vi "CS SQL Server.sql read.vi"(3 "error in (no error)":errorcluster, 4 "object":string, 5 "Data Source":string) -> (0 "error out":errorcluster, 1 "Class":string, 2 "query results":string[][](table))   [LabVIEW 2014, in "CS SQL Server.lvlib"]
doc: "This VI retrieves data associated with the BaseProcess attribute data from a DataBase via SQL (tested with MS Access).\n\nLicense Agreement:\n\nCopyright (C)\nGesellschaft für Schwerionenforschung, GSI\nPlanckstr. 1\n64291 Darmstadt\nGermany\n\nContact: D.Beck@gsi.de \n\nThis program is free software; you can redistribute it and/or modify it under the terms of the \nGNU General Public License as published by the Free Software Foundation; either version 2 of the license, or (at your option) any later version.\n\nThis program is distributed in the hope that it will be useful, but WITHOUT ANY WARRANTY; without even the implied warranty of MERCHANTABILITY or FITNESS FOR A PARTICULAR PURPOSE. See the GNU General License for more details (http://www.gnu.org).\n\nGesellschaft für Schwerionenforschung, GSI\nPlanckstr. 1, 64291 Darmstadt, Germany\nFor all questions and ideas contact: M.Richter@gsi.de, K.Poppensieker, H.Brand@gsi.de or D.Beck@gsi.de.\nLast update: 20-JUN-2002"
uses:
  CS SQL Server.lvlib
  <vilib>/addons/database/Recordset.llb/Rec Destroy - Connection.vi
  <vilib>/addons/database/Recordset.llb/Rec Fetch Recordset Data (R).vi
  <vilib>/addons/database/Connection.llb/Conn Execute.vi
  <vilib>/addons/database/Connection.llb/DB Tools Open Connec (String).vi
  <vilib>/addons/database/_DB Variant To Data/Database Variant To Data.xnode
  <vilib>/addons/database/NI_Database_API.lvlib
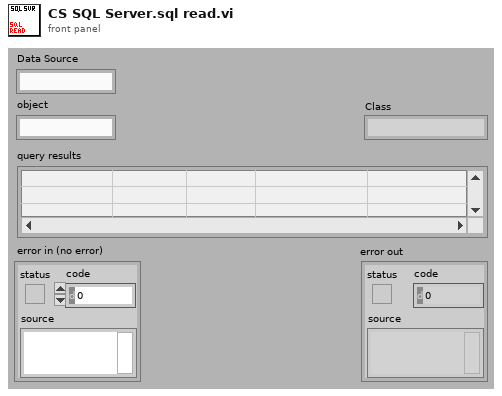
[diagram p1: front panel]
types:
  T1 = typedef "NI_Database_API.lvlib/Conn ObjectReference.ctl" = refnum<k1>
  T2 = typedef "NI_Database_API.lvlib/Rec ObjectReference.ctl" = refnum<k1>
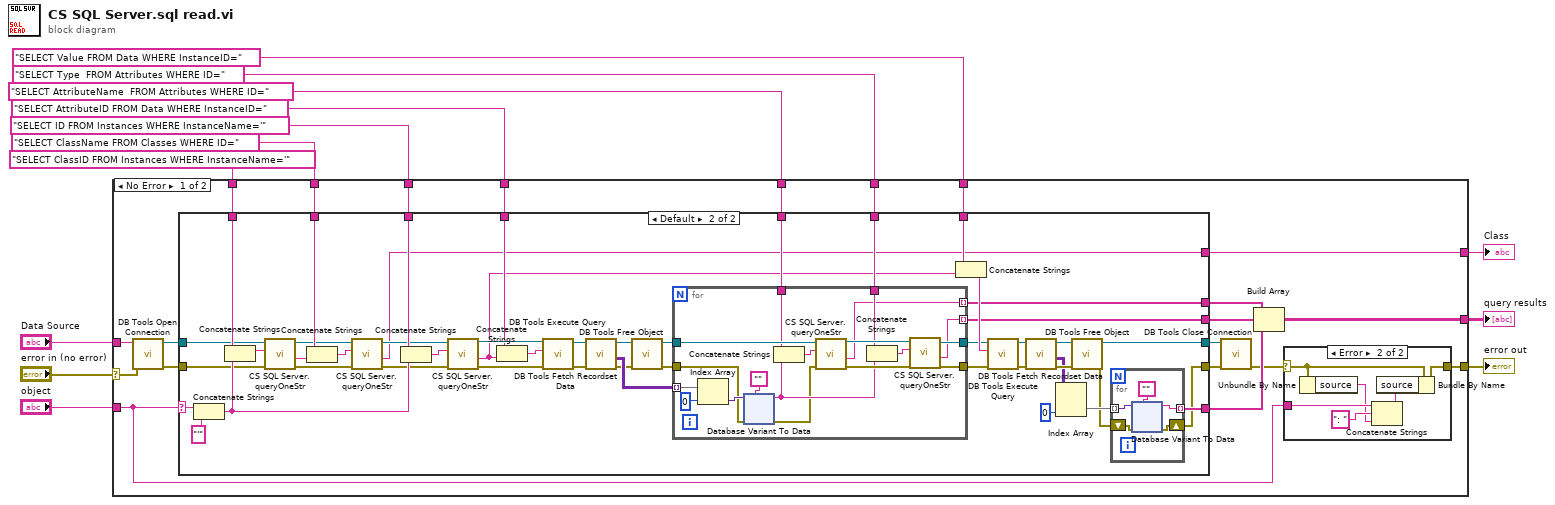
[diagram p0: block diagram]
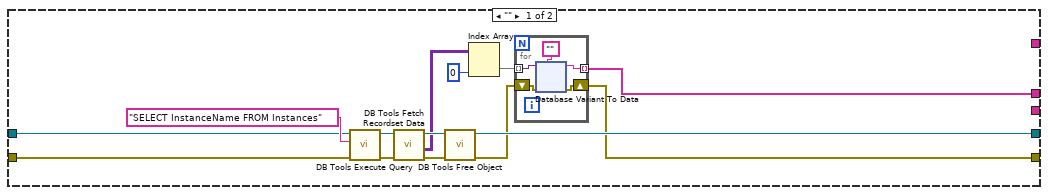
[diagram p3: hidden frame]
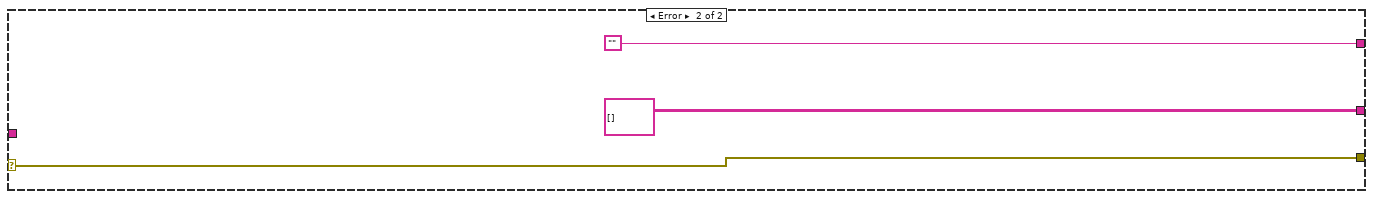
[diagram p4: hidden frame]
diagram:
  n1 = case shown="No Error" "error in (no error)" {
    selector: "error in (no error)" -> [w30 w230]
    tunnel: "Data Source" -> [w19 _]
    tunnel: "SELECT ID FROM Instances WHERE InstanceName='" -> [w27 _]
    tunnel: "object" -> [w20 _]
    tunnel: "SELECT AttributeID FROM Data WHERE InstanceID=" -> [w34 _]
    tunnel: "SELECT AttributeName  FROM Attributes WHERE ID=" ("SQL statement") -> [w33 _]
    tunnel: "SELECT Value FROM Data WHERE InstanceID=" -> [w32 _]
    tunnel: [w14 string[][] []] -> w7
    tunnel: [w16 w230] -> w6
    tunnel: "SELECT ClassID FROM Instances WHERE InstanceName='" -> [w26 _]
    tunnel: "SELECT ClassName FROM Classes WHERE ID=" -> [w25 _]
    tunnel: [w24 ""] -> w2
    tunnel: "SELECT Type  FROM Attributes WHERE ID=" ("SQL statement") -> [w23 _]
    frame No Error {
      n2 = call-poly <vilib>:"DB Tools Open Connection.vi"("error in (no error)"=w30, "connection information"=w19) -> ("error out"=w28:errorcluster, "connection reference"=w29:T1)  [unwired: 6 in]
      n3 = case shown="Default" w20 {
        selector: w20 -> [_ w118]
        tunnel: w34 -> [_ w137]
        tunnel: w33 -> [_ w135]
        tunnel: w32 -> [_ w133]
        tunnel: [_ w95] -> w31
        tunnel: [w47 w97] -> w15
        tunnel: w29 -> [w54 w117]
        tunnel: w28 -> [w52 w115]
        tunnel: w27 -> [_ w129]
        tunnel: w26 -> [_ w126]
        tunnel: w25 -> [_ w123]
        tunnel: [_ w111] -> w24
        tunnel: w23 -> [_ w121]
        tunnel: [w44 w120] -> w22
        tunnel: [_ w119] -> w21
        tunnel: [w42 w93] -> w18
        frame "" {
          n4 = call-poly <vilib>:"DB Tools Execute Query.vi"("error in (no error)"=w52, "SQL query"="SELECT InstanceName FROM Instances", "connection reference"=w54) -> ("error out"=w49:errorcluster, "recordset reference"=w53:T2)  [unwired: 5 in]
          n5 = call-poly <vilib>:"DB Tools Fetch Recordset Data.vi"("error in (no error)"=w49, "recordset reference"=w53) -> ("error out"=w46:errorcluster, "recordset data"=w48:variant[][], "recordset reference out"=w50:T2)  [unwired: 3 in]
          n6 = call-poly <vilib>:"DB Tools Free Object.vi"("error in (no error)"=w46, "recordset reference"=w50) -> ("error out"=w43:errorcluster, "connection reference"=w47:T1)  [unwired: 8 in]
          n7 = Index Array(array=w48, index (col)=0 ("disabled index (col)")) -> (element=w45:variant[])  [unwired: 1 in]
          n8 = for {
            tunnel: w45 -> [w59] mode=indexing
            tunnel: [w58] -> w44 mode=indexing
            shift-right: [w56] -> w42
            shift-left: w43 -> [w57]
            n9 = xnode "Database Variant To Data"("database variant"=w59, "error in (no error)"=w57, "type"="") -> ("data"=w58:string, "error out"=w56:errorcluster)
          }
        }
        frame Default {
          n10 = Concatenate Strings(w118, "'" ("Substring")) -> (w127:string)
          n11 = Concatenate Strings(w126, w127) -> (w116:string)
          n12 = call "CS SQL Server.queryOneStr.vi"("error in (no error)"=w115, "SQL query"=w116, "connection reference"=w117) -> ("error out"=w113:errorcluster, "Query result"=w112:string, "connection reference out"=w114:T1)  [unwired: 6 in]
          n13 = Concatenate Strings(w123, w112) -> (w122:string)
          n14 = call "CS SQL Server.queryOneStr.vi"("error in (no error)"=w113, "SQL query"=w122, "connection reference"=w114) -> ("error out"=w124:errorcluster, "Query result"=w111:string, "connection reference out"=w125:T1)  [unwired: 6 in]
          n15 = Concatenate Strings(w129, w127) -> (w128:string)
          n16 = call "CS SQL Server.queryOneStr.vi"("error in (no error)"=w124, "SQL query"=w128, "connection reference"=w125) -> ("error out"=w139:errorcluster, "Query result"=w110:string, "connection reference out"=w138:T1)  [unwired: 6 in]
          n17 = Concatenate Strings(w137, w110) -> (w136:string)
          n18 = call-poly <vilib>:"DB Tools Execute Query.vi"("error in (no error)"=w139, "SQL query"=w136, "connection reference"=w138) -> ("error out"=w109:errorcluster, "recordset reference"=w108:T2)  [unwired: 5 in]
          n19 = call-poly <vilib>:"DB Tools Fetch Recordset Data.vi"("error in (no error)"=w109, "recordset reference"=w108) -> ("error out"=w106:errorcluster, "recordset data"=w107:variant[][], "recordset reference out"=w105:T2)  [unwired: 3 in]
          n20 = call-poly <vilib>:"DB Tools Free Object.vi"("error in (no error)"=w106, "recordset reference"=w105) -> ("error out"=w103:errorcluster, "connection reference"=w104:T1)  [unwired: 8 in]
          n21 = for {
            tunnel: w104 -> [w195]
            tunnel: w103 -> [w179]
            tunnel: w107 -> [w193] mode=indexing
            tunnel: w135 -> [w194]
            tunnel: [w181] -> w120 mode=indexing
            tunnel: [w187] -> w132
            tunnel: [w185] -> w131
            tunnel: w121 -> [w186]
            tunnel: [w180] -> w119 mode=indexing
            n22 = Index Array(array=w193, index=0 ("Index (row)")) -> (element=w184:variant)
            n23 = xnode "Database Variant To Data"("database variant"=w184, "error in (no error)"=w179, "type"="") -> ("data"=w182:string, "error out"=w178:errorcluster)
            n24 = Concatenate Strings(w194, w182) -> (w191:string)
            n25 = call "CS SQL Server.queryOneStr.vi"("error in (no error)"=w178, "SQL query"=w191, "connection reference"=w195) -> ("error out"=w188:errorcluster, "Query result"=w181:string, "connection reference out"=w189:T1)  [unwired: 6 in]
            n26 = Concatenate Strings(w186, w182) -> (w190:string)
            n27 = call "CS SQL Server.queryOneStr.vi"("error in (no error)"=w188, "SQL query"=w190, "connection reference"=w189) -> ("error out"=w185:errorcluster, "Query result"=w180:string, "connection reference out"=w187:T1)  [unwired: 6 in]
          }
          n28 = Concatenate Strings(w133, w110) -> (w134:string)
          n29 = call-poly <vilib>:"DB Tools Execute Query.vi"("error in (no error)"=w131, "SQL query"=w134, "connection reference"=w132) -> ("error out"=w100:errorcluster, "recordset reference"=w101:T2)  [unwired: 5 in]
          n30 = call-poly <vilib>:"DB Tools Fetch Recordset Data.vi"("error in (no error)"=w100, "recordset reference"=w101) -> ("error out"=w99:errorcluster, "recordset data"=w98:variant[][], "recordset reference out"=w102:T2)  [unwired: 3 in]
          n31 = Index Array(array=w98, index (col)=0 ("Disabled Index (col)")) -> (element=w96:variant[])  [unwired: 1 in]
          n32 = call-poly <vilib>:"DB Tools Free Object.vi"("error in (no error)"=w99, "recordset reference"=w102) -> ("error out"=w94:errorcluster, "connection reference"=w97:T1)  [unwired: 8 in]
          n33 = for {
            tunnel: w96 -> [w144] mode=indexing
            tunnel: [w143] -> w95 mode=indexing
            shift-right: [w141] -> w93
            shift-left: w94 -> [w142]
            n34 = xnode "Database Variant To Data"("database variant"=w144, "error in (no error)"=w142, "type"="") -> ("data"=w143:string, "error out"=w141:errorcluster)
          }
        }
      }
      n35 = call <vilib>:"DB Tools Close Connection.vi"("error in (no error)"=w18, "connection reference"=w15) -> ("error out"=w17:errorcluster)  [unwired: 5 in]
      n36 = Build Array(w22, w21, w31) -> (w14:string[][])
      n37 = case shown="Error" w17 {
        selector: w17 -> [w35 w38]
        tunnel: [w35 w36] -> w16
        tunnel: w20 -> [_ w39]
        frame No Error {
        }
        frame Error {
          n38 = Unbundle By Name(w38) -> ("source"=w37:string)
          n39 = Concatenate Strings(w39, ": " ("string"), w37) -> (w41:string)
          n40 = Bundle By Name(cluster=w38, "source"=w41) -> (w36:errorcluster)
        }
      }
    }
    frame Error {
    }
  }
  "query results" <- w7
  "error out" <- w6
  "Class" <- w2
